vi "SCStandAlone.vi"() -> ()   [LabVIEW 2014]
uses:
  Controls/heinzingerSelect.ctl
  Controls/DacState.ctl
  Controls/triggerTypes.ctl
  <vilib>/rvi/Emulation/niFpgaGetClockAttributes.vi
  <vilib>/rvi/Emulation/niFpgaSctlEmulationGetInTimedLoop.vi
  <vilib>/rvi/Emulation/niFpgaEmulationReportErrorSimple.vi
  <vilib>/rvi/Emulation/niFpgaCriticalErrorInLSC.vi
  DAC/Code/FPGA SPI_Globals.vi
  HeinzingerControl/heinzingerControlGlobals.vi
panel:
  out "DacState":T1
  out "actDACRegister":u32=1572792 caption="actRegister" format="%024b"
  in  "setDACRegister":u32=1048576 format="%024b"
  in  "DacStateCmdByHost":T1
  in  "postAccOffsetVoltControl":T2
  out "postAccOffsetVoltState":T2
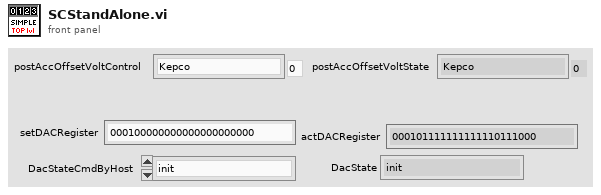
[diagram p1: front panel]
types:
  T1 = typedef "DacState.ctl" = enum16{"init", "idle", "setVolt", "error"}
  T2 = typedef "heinzingerSelect.ctl" = enum8{"Kepco", "Heinzinger0", "Heinzinger1", "Heinzinger2", "loading"}
  T3 = typedef "triggerTypes.ctl" = enum16{"noTrigger", "singleHitDelay", "singleHit"}
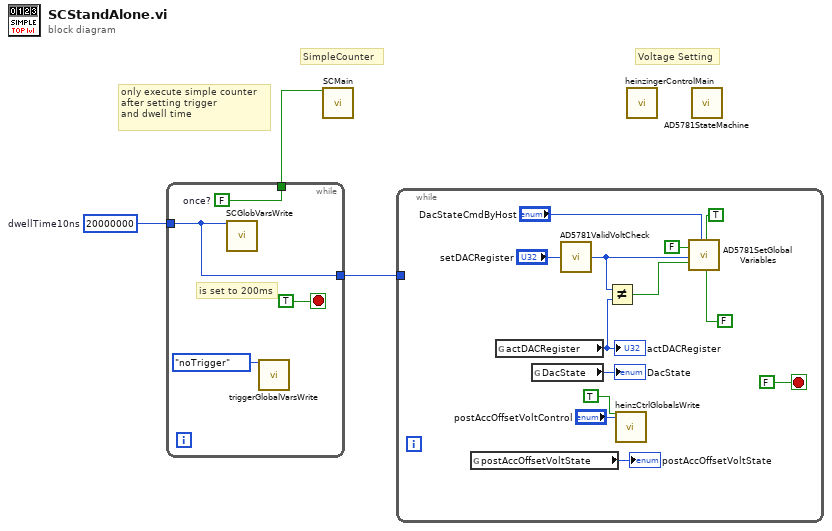
[diagram p0: block diagram]
diagram:
  w3 = u32 20000000  # dwellTime10ns
  # "only execute simple counter\nafter setting trigger\nand dwell time"
  # "Voltage Setting"
  # "SimpleCounter"
  n1 = while {
    tunnel: w3 -> [w5]
    tunnel: [w7] -> w2
    tunnel: [w5] -> w1
    stop <- TRUE stop-if-true
    w7 = FALSE  # once?
    # "is set to 200ms"
    n2 = call "SCGlobVarsWrite.vi"("dwellTime10ns"=w5) -> ()  [unwired: 19 in]
    n3 = call "triggerGlobalVarsWrite.vi"("triggerTypes"=triggerTypes."noTrigger") -> ()  [unwired: 19 in]
  }
  n4 = call "SCMain.vi"("once?"=w2) -> ()  [unwired: 19 in]
  n5 = while {
    tunnel: w1 -> [_]
    stop <- FALSE stop-if-true
    n6 = global read "heinzingerControlGlobals.vi" "postAccOffsetVoltState"() -> (→"postAccOffsetVoltState":T2)
    n7 = global read "FPGA SPI_Globals.vi" "actDACRegister"() -> (w16:u32)
    "actDACRegister" <- w16
    n8 = global read "FPGA SPI_Globals.vi" "DacState"() -> (→"DacState":T1)
    n9 = call "AD5781ValidVoltCheck.vi"("U32"="setDACRegister") -> ("coerced(x)"=w14:u32)  [unwired: 4 in]
    n10 = Not Equal?(x=w14, y=w16) -> (x != y?=w15:bool)
    n11 = call "heinzCtrlGlobalsWrite.vi"("w_postAccOffsetVoltControl"=TRUE, "postAccOffsetVoltControl"="postAccOffsetVoltControl") -> ()  [unwired: 26 in]
    n12 = call "AD5781SetGlobalVariables.vi"("write actDACRegister"=FALSE, "setDACRegister"=w14, "write setDACRegister"=w15, "DacStateCmdByHost"="DacStateCmdByHost", "write DacStateCmdByHost"=TRUE, "write DacState"=FALSE) -> ()  [unwired: 14 in]
  }
  n13 = call "heinzingerControlMain.vi"() -> ()  [unwired: 3 in]
  n14 = call "AD5781StateMachine.vi"() -> ()  [unwired: 12 in]
